vi "CleanUp.vi"(0 "object in":refnum<class "CoriFlowBFS1Plus.lvclass">, 5 "error in (no error)":errorcluster) -> (14 "object out":refnum<class "CoriFlowBFS1Plus.lvclass">, 19 "error out":errorcluster)   [LabVIEW 2021, in "CoriFlowBFS1Plus.lvclass"]
uses:
  CoriFlowBFS1Plus.lvclass
  CoriFlowBFS1Plus.lvclass/CoriFlowBFS1Plus.ctl
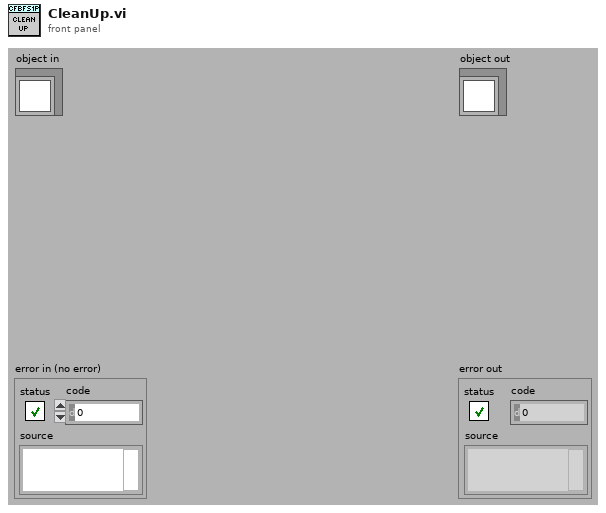
[diagram p1: front panel]
types:
  T1 = typedef "Z_BFS_type.ctl" = cluster{"VISA_Name":refnum<visa-resource-name>, "density_g_L":dbl, "Capacity":dbl, "Capacity units conversion":dbl}
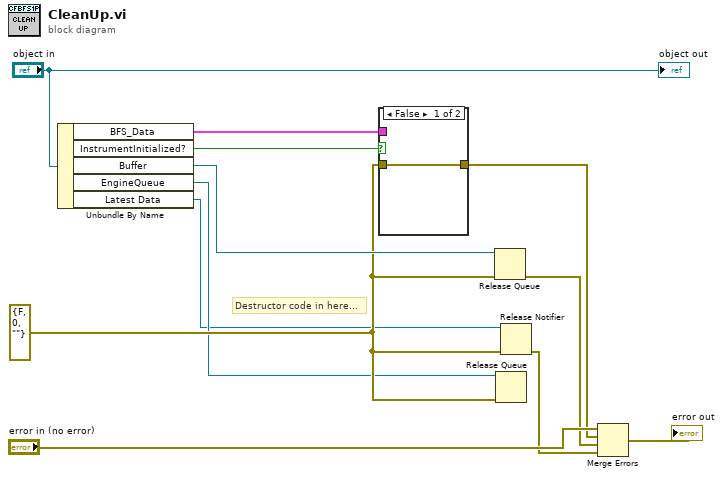
[diagram p0: block diagram]
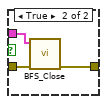
[diagram p2: hidden frame]
diagram:
  w3 = errorcluster {"status"=FALSE, "code"=0, "source"=""} ("error in (no error)")
  # "Destructor code in here..."
  n1 = Unbundle By Name("object in") -> ("BFS_Data"=w9:T1, "InstrumentInitialized?"=w7:bool, "Buffer"=w6:refnum<queue>, "EngineQueue"=w2:refnum<queue>, "Latest Data"=w1:refnum<notifier>)
  n2 = case shown="False" w7 {
    tunnel: w9 -> [_ w16]
    tunnel: w3 -> [w13 w14]
    tunnel: [w13 w15] -> w8
    frame False {
    }
    frame True {
      n3 = call "BFS_Close.vi"("error in"=w14, "BFS_In"=w16) -> ("error out"=w15:errorcluster)  [unwired: 9 in]
    }
  }
  n4 = Release Queue(queue=w6, error in (no error)=w3) -> (error out=w5:errorcluster)  [unwired: 1 in, 2 out]
  n5 = Release Queue(queue=w2, error in (no error)=w3) -> ()  [unwired: 1 in, 3 out]
  n6 = Release Notifier(notifier=w1, error in (no error)=w3) -> (error out=w4:errorcluster)  [unwired: 1 in, 2 out]
  n7 = Merge Errors("error in (no error)", w8, w5, w4) -> (→"error out":errorcluster)
  "object out" <- "object in"
